vi "Property Control.vi"() -> ()   [LabVIEW 2019, in "LSS.lvlib"]
doc: "This example demonstrates how to use the Property Control Engine paired with LSS strings to minimize the amount of LabVIEW code that must be written in order to control the style of a user interface."
uses:
  LSS.lvlib
panel:
  in  "Setpoint 2":dbl(knob) scale=0.0..10.0
  in  "Setpoint":dbl(knob) scale=0.0..10.0
  out "Warning":string="WARNING\nWARNING"
  in  "Numeric":dbl
  in  "Change Styles":bool
  # "Since the control engine is asynchronously launched as a clone, if you abort this VI,\nthe control engine will not be aborted.  It is strongly recommended that you close \nthis VI using the \"X\" in the upper right hand corner like how a normal program \nwould close."
  # "Run this VI then play with the various controls to observe their behavior, then\nnavigate to the block diagram and observe how the code implements these\nbehaviors."
  # "Setpoint one controls it's own background\ncolor as well as the background color of the\nsplitter bar.  Take note on the block diagram\nhow no LabVIEW code was written in order\nto implement this."
  # "Setpoint 2 controls the background color of\nthe RightPane. Notice how it also changes \nthe background color of the \"Numeric\"\ncontrol.  This is because \"Numeric\" is owned\nby the \"RightPane\", and properties cascade\nin cascading style sheets.  To have a different\nstyle for the Numeric, add\n#Numeric {background-color:#somecolor}\nto the LSS on the block diagram. \n\nAlso, if both controls are above 7, then a \nwarning indicator will appear.  This is to demo\nhow multiple conditions applied within the\nsame line."
  # "Use the Change Styles button to change\nthe background color of this panel.  \nNote that if you use Setpoint 2, this \nproperty is overwritten.  This is because\nwhichever property is applied LAST is\nthe one that will be visible."
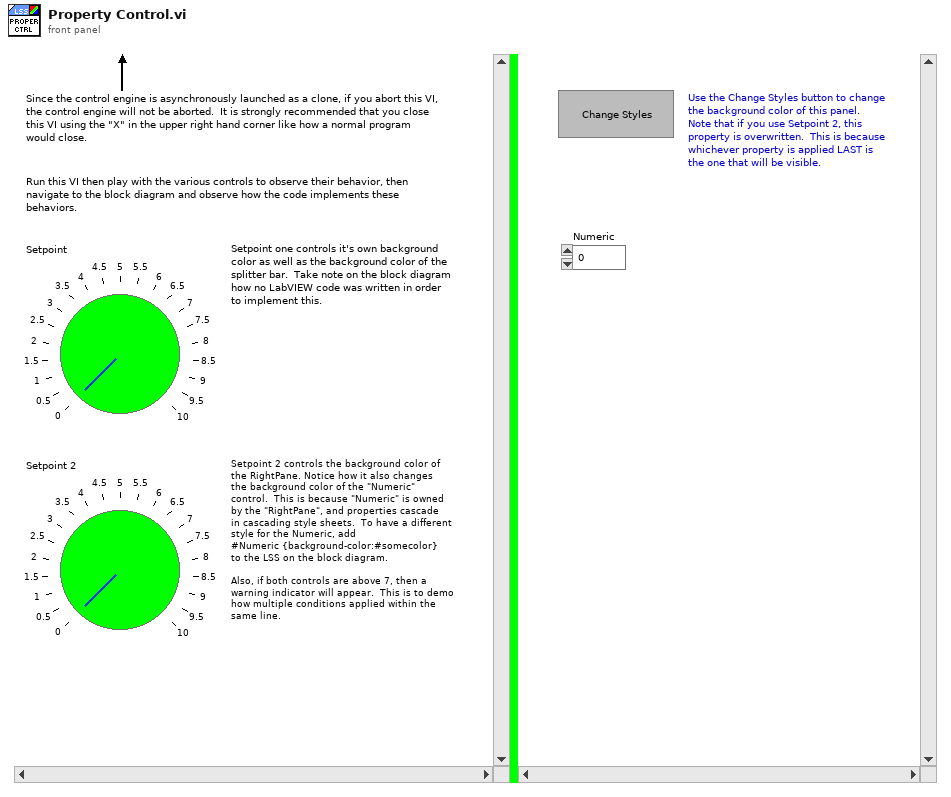
[diagram p1: front panel]
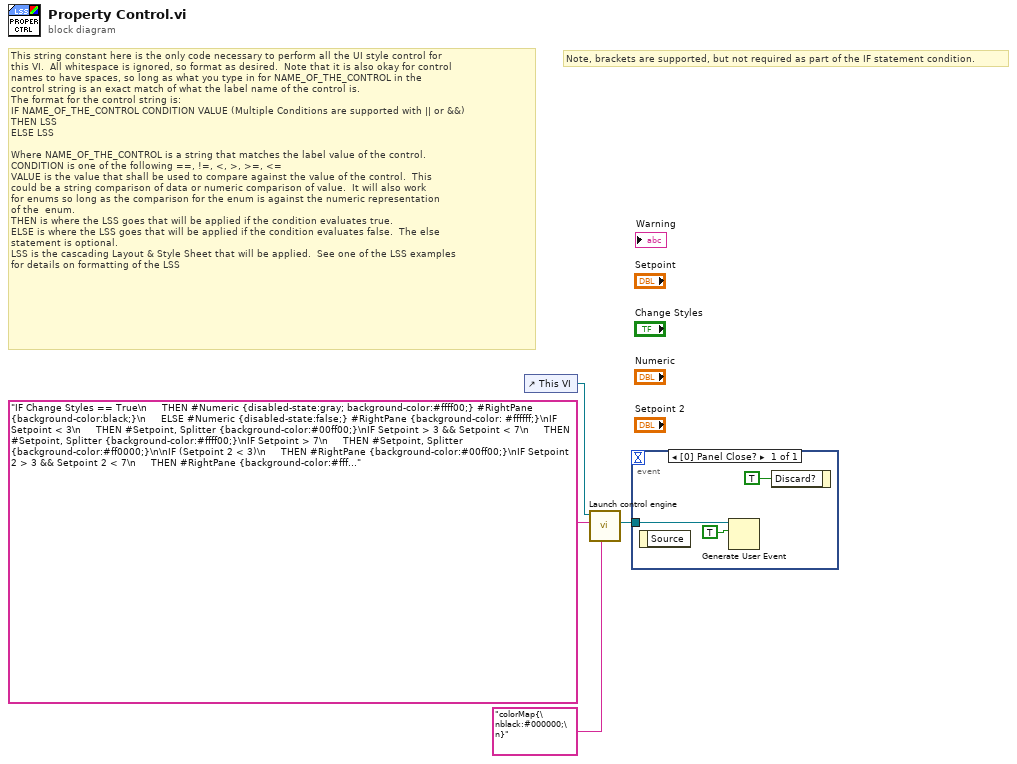
[diagram p0: block diagram]
diagram:
  # "Note, brackets are supported, but not required as part of the IF statement condition."
  # "This string constant here is the only code necessary to perform all the UI style control for \nthis VI.  All whitespace is ignored, so format as desired.  Note that it is also okay for control\nnames to have spaces, so long as what you type in for NAME_OF_THE_CONTROL in the\ncontrol string is an exact match of what the label name of the control is.\nThe format for the control string is:\nIF NAME_OF_THE_CONTROL CONDITION VALUE (Multiple Conditions are supported with || or &&)\nTHEN LSS\nELSE LSS\n\nWhere NAME_OF_THE_CONTROL is a string that matches the label value of the control.\nCONDITION is one of the following ==, !=, <, >, >=, <=\nVALUE is the value that shall be used to compare against the value of the control.  This\ncould be a string comparison of data or numeric comparison of value.  It will also work\nfor enums so long as the comparison for the enum is against the numeric representation \nof the  enum.\nTHEN is where the LSS goes that will be applied if the condition evaluates true.  \nELSE is where the LSS goes that will be applied if the condition evaluates false.  The else\nstatement is optional.\nLSS is the cascading Layout & Style Sheet that will be applied.  See one of the LSS examples\nfor details on formatting of the LSS"
  n1 = control-ref of="This VI"() -> (w4:refnum<vi>)
  n2 = call "Launch control engine.vi"("colorMap"="colorMap{\nblack:#000000;\n}", "Rules String"="IF Change Styles == True\n     THEN #Numeric {disabled-state:gray; background-color:#ffff00;} #RightPane {background-color:black;}\n     ELSE #Numeric {disabled-state:false;} #RightPane {background-color: #ffffff;}\nIF Setpoint < 3\n     THEN #Setpoint, Splitter {background-color:#00ff00;}\nIF Setpoint > 3 && Setpoint < 7\n     THEN #Setpoint, Splitter {background-color:#ffff00;}\nIF Setpoint > 7\n     THEN #Setpoint, Splitter {background-color:#ff0000;}\n\nIF (Setpoint 2 < 3)\n     THEN #RightPane {background-color:#00ff00;}\nIF Setpoint 2 > 3 && Setpoint 2 < 7\n     THEN #RightPane {background-color:#ffff00;}\nIF Setpoint 2 > 7\n     THEN #RightPane {background-color:#ff0000;}\n\nIF ((Setpoint > 7) && (Setpoint 2 > 7))\n     THEN #Warning {visible:true;}\n     ELSE #Warning {visible:false;} ", "Controlled VI"=w4) -> ("Exit event"=w3:refnum<user-event>)  [unwired: 6 in, 2 out]
  n3 = event shown="[0] Panel Close?" {
    selector: _ -> [_]
    dyn-events: _ -> [_]
    timeout: _ -> [_]
    tunnel: w3 -> [w7]
    event Panel Close? {
      n4 = event-data() -> ()  [unwired: 1 in, 1 out]
      n5 = Generate User Event(user event=w7, event data cluster=TRUE ("event data")) -> ()  [unwired: 2 in, 2 out]
      n6 = event-data("Discard?"=TRUE) -> ()  [unwired: 1 in, 1 out]
    }
  }
